vi "RC_Client.vi"(8 "error in (no error)":errorcluster, 10 "ID":i32, 11 "RC Type":T1) -> (0 "error out":errorcluster)   [LabVIEW 2019, in "RemoteControl.lvclass"]
uses:
  RemoteControl.lvclass
  Typedefs/RC Com Type--enum.ctl
  d5fabe2d-a353-4028-afbd-9badd668dfe0.vi
  86a5ece5-b561-413e-9f09-d5d31fd20f43.vi
  65f66a04-8a0d-4a92-b0ec-22ee31523ff5.vi
  d5fabe2d-a353-4028-afbd-9badd668dfe0.vi/c4a56862-488f-41dc-a0a5-e5ee077bd9ca.vi
  86a5ece5-b561-413e-9f09-d5d31fd20f43.vi/d95e8ff3-4598-449c-975a-e92d1b076826.vi
  65f66a04-8a0d-4a92-b0ec-22ee31523ff5.vi/241116c3-eed1-40cd-b5db-cbb2db086cd1.vi
  <vilib>/Utility/LVClass/Get LV Class Name.vi
  <vilib>/JDP Science/JSONtext/JSON text to Variant.vi
  <userlib>/_OpenG.lib/numeric/numeric.llb/Random Number Within Range - I32__ogtk.vi
  <userlib>/_OpenG.lib/error/error.llb/Filter Error Codes (Array)__ogtk.vi
  <vilib>/JDP Science/JSONtext/LVClass Serializer/JSONtext LVClass Serializer.lvclass
panel:
  in  "milliseconds to wait":u32
  out "time (1 message) (s)":dbl
  out "startup time (s)":dbl
  out "messages/s":dbl
  in  "remote port":u16=6341
  in  "address":string
  out "Response":string
  out "Messages":i32
  in  "Stop":bool
  out "Command reponse":string
  out "Command":string
  out "meta data\n(available commands)":string
  # "CLIENT (API)"
  # "Connection info"
  # "Message Sent"
  # "Message Received"
  # "Metrics"
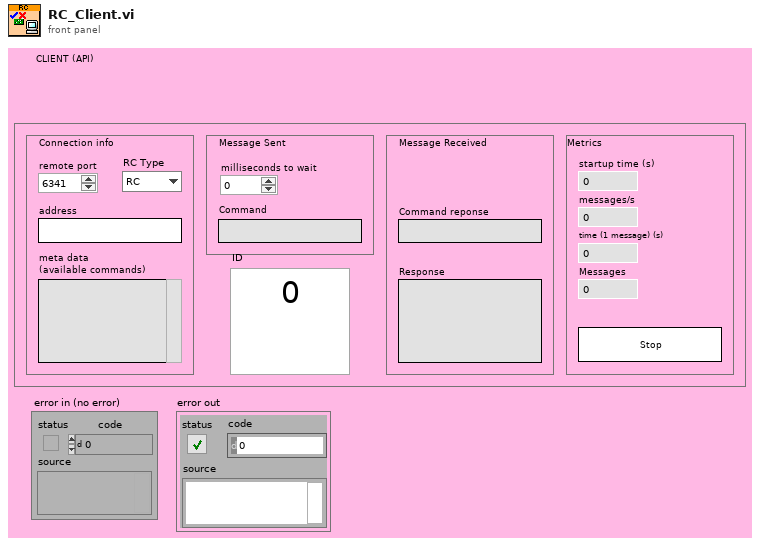
[diagram p1: front panel]
types:
  T1 = typedef "RemoteControl.lvclass/RC Com Type--enum.ctl" = enum16{"RC", "STM", "ZMQ"}
  T2 = cluster{"Command out":string, "Data out":string, string}
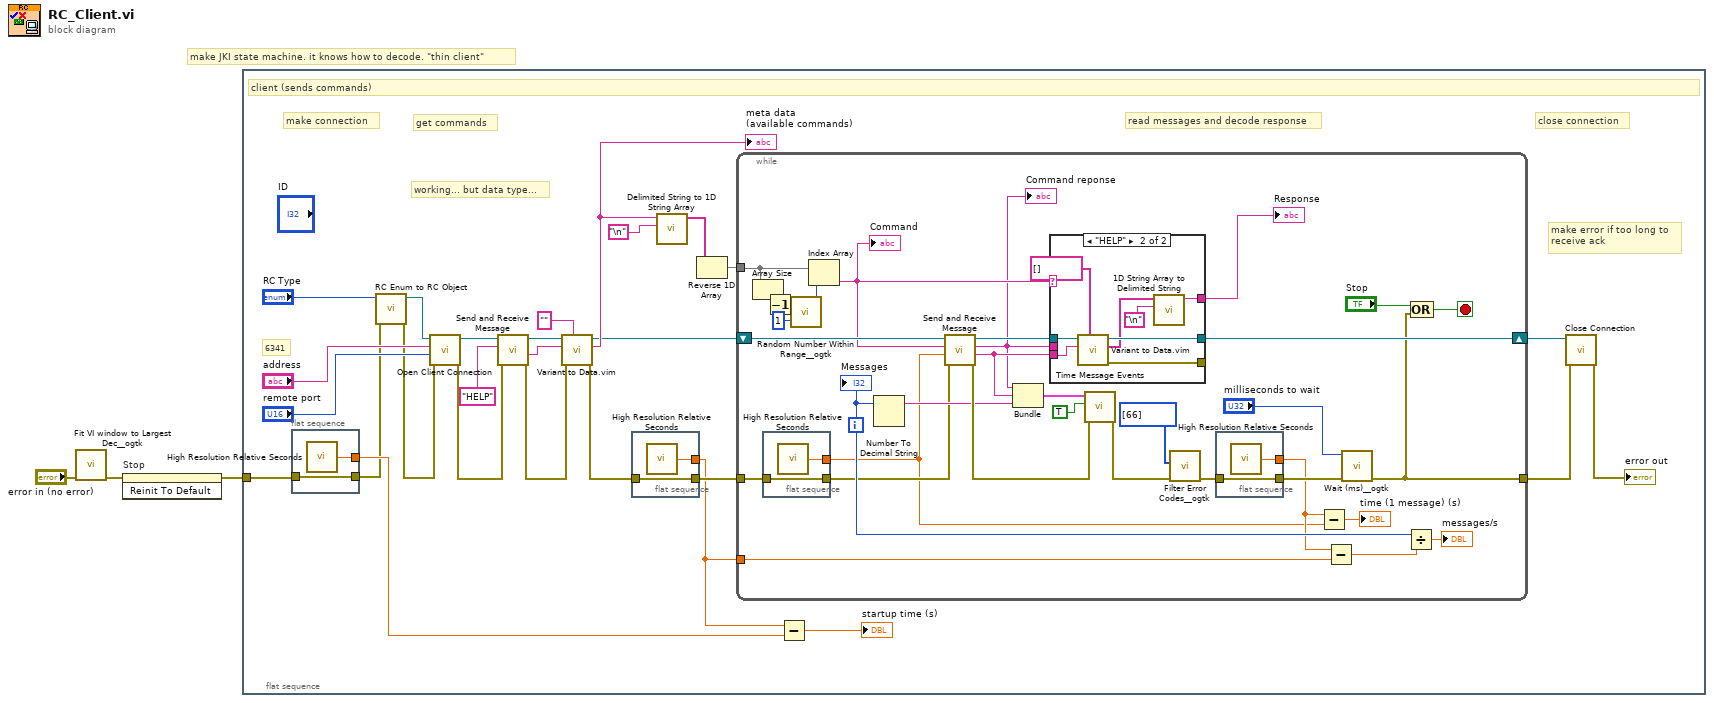
[diagram p0: block diagram]
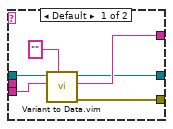
[diagram p2: hidden frame]
diagram:
  # "make JKI state machine. it knows how to decode. \"thin client\""
  n1 = call <userlib>:"Fit VI window to Largest Dec__ogtk.vi"("error in (no error)"="error in (no error)") -> ("error out"=w3:errorcluster)  [unwired: 5 in, 1 out]
  n2 = invoke on="Stop" class="Bool" method="Reinit To Default"(error in=w3) -> (error out=w2:errorcluster)  [unwired: 2 in, 2 out]
  n3 = flat-sequence {
    tunnel: w2 -> [w16]
    frame #0 {
      # "working... but data type..."
      # "close connection"
      # "read messages and decode response"
      # "get commands"
      # "make connection"
      # "6341"
      # "make error if too long to\nreceive ack"
      # "client (sends commands)"
      n4 = flat-sequence {
        tunnel: [w31] -> w13
        tunnel: [w32] -> w15
        tunnel: w16 -> [w31]
        frame #0 {
          n5 = call <vilib>:"High Resolution Relative Seconds.vi"() -> ("relative seconds"=w32:dbl)
        }
      }
      n6 = call "RC Enum to RC Object.vi"("error in (no error)"=w13, "RC Type"="RC Type") -> ("error out"=w12:errorcluster, "RemoteControl out"=w19:refnum<class "RemoteControl.lvclass">)  [unwired: 8 in]
      n7 = call-dynamic "Open Client Connection.vi"("error in (no error)"=w12, "Port"="remote port", "address"="address", "RemoteControl in"=w19) -> ("error out"=w21:errorcluster, "RemoteControl out"=w20:refnum<class "RemoteControl.lvclass">)  [unwired: 6 in]
      n8 = call-dynamic "Send and Receive Message.vi"("error in (no error)"=w21, "Command"="HELP", "RemoteControl in"=w20) -> ("error out"=w5:errorcluster, "Data out"=w10:string, "RemoteControl out"=w8:refnum<class "RemoteControl.lvclass">)  [unwired: 5 in, 1 out]
      n9 = call "Variant to Data.vim"("Data Type"="", "error in (no error)"=w5, "Data in"=w10, "RemoteControl in"=w8) -> ("error out"=w4:errorcluster, "Data out"=w7:string, "RemoteControl out"=w6:refnum<class "RemoteControl.lvclass">)  [unwired: 5 in]
      "meta data\n(available commands)" <- w7
      n10 = flat-sequence {
        tunnel: [w33] -> w25
        tunnel: [w34] -> w22
        tunnel: w4 -> [w33]
        frame #0 {
          n11 = call <vilib>:"High Resolution Relative Seconds.vi"() -> ("relative seconds"=w34:dbl)
        }
      }
      n12 = call <vilib>:"Delimited String to 1D String Array.vi"("delimiter"="\n", "delimited string"=w7) -> ("string array"=w11:string[])  [unwired: 9 in]
      n13 = Reverse 1D Array(array=w11) -> (reversed array=w26:string[])
      n14 = while {
        tunnel: [w45] -> w30
        tunnel: w25 -> [w38]
        tunnel: w26 -> [w58]
        tunnel: w22 -> [w53]
        shift-right: [w48] -> w29
        shift-left: w6 -> [w66]
        i -> [w44]
        stop <- w43 stop-if-true
        n15 = Array Size(array=w58) -> (size(s)=w59:i32)
        n16 = flat-sequence {
          tunnel: [w68] -> w37
          tunnel: [w69] -> w36
          tunnel: w38 -> [w68]
          frame #0 {
            n17 = call <vilib>:"High Resolution Relative Seconds.vi"() -> ("relative seconds"=w69:dbl)
          }
        }
        n18 = Decrement(x=w59) -> (x-1=w57:i32)
        n19 = call-poly <userlib>:"Random Number Within Range__ogtk.vi"("High"=w57, "Low"=1) -> ("Random Number"=w61:i32)  [unwired: 3 in]
        n20 = Index Array(array=w58, index=w61) -> (element=w46:string)
        "Command" <- w46
        n21 = Number To Decimal String(number=w44) -> (decimal integer string=w47:string)  [unwired: 1 in]
        n22 = call-dynamic "Send and Receive Message.vi"("error in (no error)"=w37, "Data"=w36, "Command"=w46, "RemoteControl in"=w66) -> ("error out"=w56:errorcluster, "Data out"=w49:string, "Command out"=w35:string, "RemoteControl out"=w50:refnum<class "RemoteControl.lvclass">)  [unwired: 4 in]
        "Command reponse" <- w35
        n23 = Bundle("Command out"=w35, "Data out"=w49, w47) -> (w64:T2)  [unwired: 1 in]
        n24 = case shown="\"HELP\"" w46 {
          tunnel: [w74 w85] -> w51
          tunnel: w50 -> [w76 w83]
          tunnel: w49 -> [w75 w80]
          tunnel: [w72 w82] -> w48
          tunnel: [w73 w78] -> _
          tunnel: w35 -> [_ _]
          frame Default {
            n25 = call "Variant to Data.vim"("Data Type"="", "Data in"=w75, "RemoteControl in"=w76) -> ("error out"=w73:errorcluster, "Data out"=w74:string, "RemoteControl out"=w72:refnum<class "RemoteControl.lvclass">)  [unwired: 6 in]
          }
          frame "HELP" {
            n26 = call "Variant to Data.vim"("Data Type"=string[] [], "Data in"=w80, "RemoteControl in"=w83) -> ("error out"=w78:errorcluster, "Data out"=w79:string[], "RemoteControl out"=w82:refnum<class "RemoteControl.lvclass">)  [unwired: 6 in]
            n27 = call <vilib>:"1D String Array to Delimited String.vi"("delimiter"="\n", "string array"=w79) -> ("delimited string"=w85:string)  [unwired: 9 in]
          }
        }
        "Response" <- w51
        n28 = call "Time Message Events.vi"("error in (no error)"=w56, "Debug Mode"=TRUE, "Message in"=w64) -> ("error out"=w52:errorcluster)  [unwired: 6 in, 2 out]
        n29 = call-poly <userlib>:"Filter Error Codes__ogtk.vi"("Error In"=w52, "Error Codes to Filter"=i32[] [66]) -> ("Error Out"=w42:errorcluster)  [unwired: 7 in, 2 out]
        n30 = flat-sequence {
          tunnel: [w70] -> w41
          tunnel: [w71] -> w40
          tunnel: w42 -> [w70]
          frame #0 {
            n31 = call <vilib>:"High Resolution Relative Seconds.vi"() -> ("relative seconds"=w71:dbl)
          }
        }
        n32 = Subtract(x=w40, y=w36) -> (x-y=→"time (1 message) (s)":dbl)
        n33 = Subtract(x=w40, y=w53) -> (x-y=w39:dbl)
        n34 = call <userlib>:"Wait (ms)__ogtk.vi"("error in (no error)"=w41, "milliseconds to wait"="milliseconds to wait") -> ("error out"=w45:errorcluster)  [unwired: 8 in, 1 out]
        n35 = Divide(x=w44, y=w39) -> (x/y=→"messages/s":dbl)
        n36 = Compound Arithmetic op=OR("Stop", w45) -> (w43:bool)
        "Messages" <- w44
      }
      n37 = Subtract(x=w22, y=w15) -> (x-y=→"startup time (s)":dbl)
      n38 = call-dynamic "Close Connection.vi"("error in (no error)"=w30, "RemoteControl in"=w29) -> ("error out"=→"error out":errorcluster)  [unwired: 8 in, 1 out]
    }
  }
